vi "case_run_gcode.vi"(7 "Main VI reference":refnum<vi>, 8 "error in (no error)":errorcluster, 9 "queue in":refnum<queue>, 10 "message cluster":T1, 11 "VISA resource name in":refnum<visa-resource-name>) -> (0 "error out":errorcluster, 3 "VISA Refnum out":refnum<visa-resource-name>)   [LabVIEW 2020]
uses:
  controls/message cluster.ctl
  61505d1a-5fdc-4f30-b844-89a9ac4bb67f.vi
  57428757-8657-4fb4-91ae-6f4533166e6c.vi
  cfd530e4-09b9-4820-a8f0-e9bb48730c15.vi
  <instrlib>/Marlin Instrument Driver/Marlin Instrument Driver.lvlib
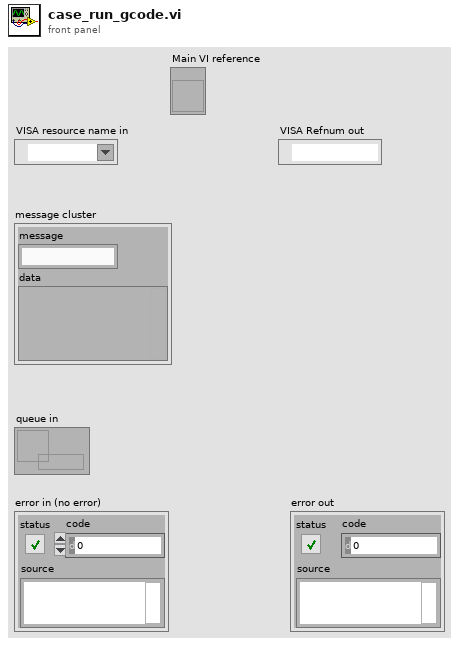
[diagram p1: front panel]
types:
  T1 = typedef "message cluster.ctl" = cluster{"message":string, "data":variant}
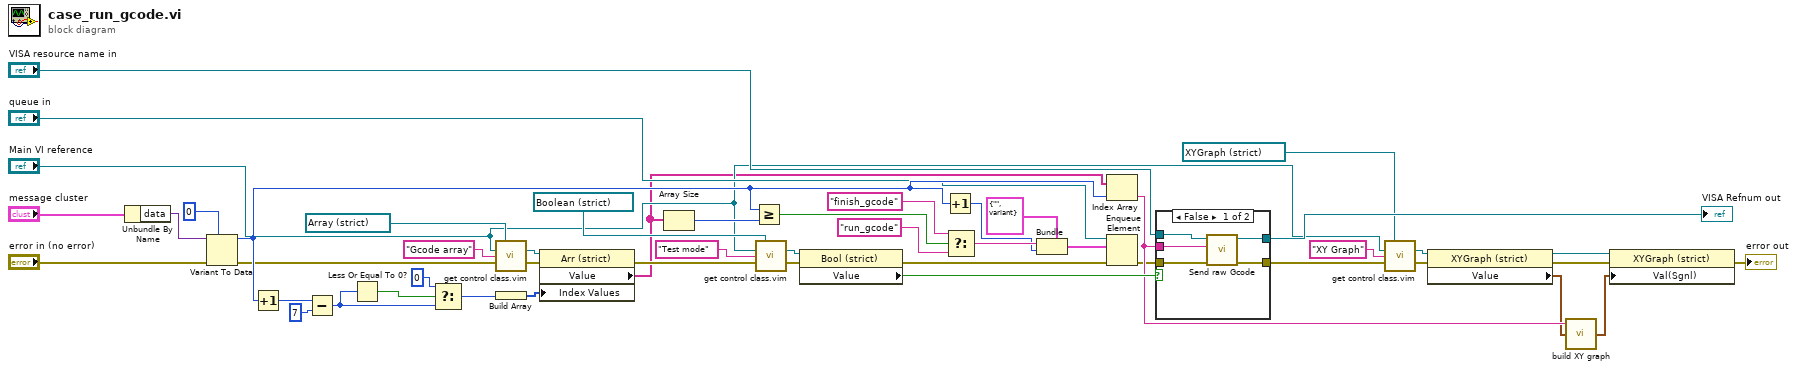
[diagram p0: block diagram]
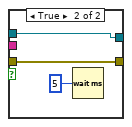
[diagram p2: hidden frame]
diagram:
  n1 = Unbundle By Name("message cluster") -> ("data"=w25:variant)
  n2 = Variant To Data(error in="error in (no error)", type=0, Variant=w25) -> (data=w41:i32, error out=w20:errorcluster)
  n3 = Increment(x=w41) -> (x+1=w42:i32)
  n4 = Subtract(x=w42, y=7) -> (x-y=w45:i32)
  n5 = Less Or Equal To 0?(x=w45) -> (x <= 0?=w44:bool)
  n6 = Select(t=0, s=w44, f=w45) -> (s? t:f=w47:i32)
  n7 = call "get control class.vim"("Control class"=refnum<vi> refnum ("Gcode array"), "Main VI reference"="Main VI reference", "Label"="Gcode array", "error in (no error)"=w20) -> ("Control out"=w22:refnum<vi>, "error out"=w21:errorcluster)  [unwired: 10 in]
  n8 = Build Array(w47) -> (w48:i32[])
  n9 = property on="Property Node" class="Arr (strict)"(reference=w22, error in=w21, "Index Values"=w48) -> (error out=w17:errorcluster, "Value"=w1:string[])  [unwired: 1 out]
  n10 = Array Size(array=w1) -> (size(s)=w35:i32)
  n11 = Greater Or Equal?(x=w41, y=w35) -> (x >= y?=w36:bool)
  n12 = call "get control class.vim"("Control class"=refnum<vi> refnum ("Test mode"), "Main VI reference"="Main VI reference", "Label"="Test mode", "error in (no error)"=w17) -> ("Control out"=w16:refnum<vi>, "error out"=w15:errorcluster)  [unwired: 10 in]
  n13 = property on="Property Node" class="Bool (strict)"(reference=w16, error in=w15) -> (error out=w13:errorcluster, "Value"=w49:bool)  [unwired: 1 out]
  n14 = Increment(x=w41) -> (x+1=w34:i32)
  n15 = Select(t="finish_gcode" ("message"), s=w36, f="run_gcode" ("message")) -> (s? t:f=w39:string)
  n16 = Bundle(cluster=T1 {"message"="", "data"=variant} ("element"), "message"=w39, "data"=w34) -> (w32:T1)
  n17 = Index Array(array=w1, index=w41) -> (element=w40:string)
  n18 = Enqueue Element(queue="queue in", element=w32, error in (no error)=w13) -> (error out=w14:errorcluster)  [unwired: 1 in, 2 out]
  n19 = case shown="False" w49 {
    tunnel: "VISA resource name in" -> [w54 w57]
    tunnel: [w53 w57] -> w30
    tunnel: w40 -> [w52 _]
    tunnel: w14 -> [w51 w55]
    tunnel: [w50 w55] -> w4
    frame False {
      n20 = call <instrlib>:"Send raw Gcode.vi"("error in (no error)"=w51, "Gcode"=w52, "VISA resource name"=w54) -> ("error out"=w50:errorcluster, "VISA resource name out"=w53:refnum<visa-resource-name>)  [unwired: 5 in, 2 out]
    }
    frame True {
      n21 = Wait (ms)(milliseconds to wait=u32 5) -> ()  [unwired: 1 out]
    }
  }
  "VISA Refnum out" <- w30
  n22 = call "get control class.vim"("Control class"=refnum<vi> refnum ("XY Graph"), "Main VI reference"="Main VI reference", "Label"="XY Graph", "error in (no error)"=w4) -> ("Control out"=w9:refnum<vi>, "error out"=w8:errorcluster)  [unwired: 10 in]
  n23 = property class="XYGraph (strict)"(reference=w9, error in=w8) -> (reference out=w6:refnum<vi>, error out=w3:errorcluster, "Value"=w7:cluster{"X":dbl, "Y":dbl}[])
  n24 = call "build XY graph.vi"("Gcode line"=w40, "XY Graph in"=w7) -> ("XY Graph out"=w5:cluster{"X":dbl, "Y":dbl}[])  [unwired: 5 in]
  n25 = property class="XYGraph (strict)"(reference=w6, error in=w3, "Val(Sgnl)"=w5) -> (error out=→"error out":errorcluster)  [unwired: 1 out]
